vi "changeFWposAcq.vi"(0 "FW pos":u8, 1 "FWhandle":u32) -> ()   [LabVIEW 2015]
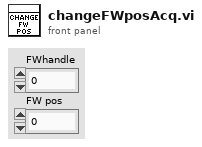
[diagram p1: front panel]
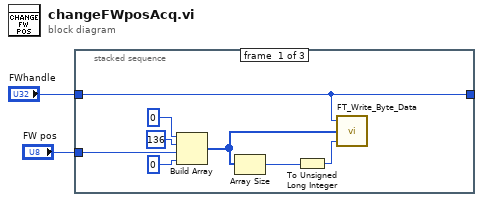
[diagram p0: block diagram]
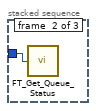
[diagram p2: hidden frame]
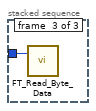
[diagram p3: hidden frame]
diagram:
  n1 = stacked-sequence {
    tunnel: "FWhandle" -> [w4 w11 w12]
    tunnel: [w4 _ _] -> _
    tunnel: "FW pos" -> [w3 _ _]
    frame #0 {
      n2 = Build Array(u8 0 ("element"), u8 136 ("element"), w3, u8 0 ("element")) -> (w10:u8[])
      n3 = Array Size(array=w10) -> (size(s)=w8:i32)
      n4 = To Unsigned Long Integer(number=w8) -> (unsigned 32bit integer=w9:u32)
      n5 = call "FT_Write_Byte_Data.vi"("Bytes To Write"=w9, "Buffer"=w10, "Handle"=w4) -> ()  [unwired: 2 out]
    }
    frame #1 {
      n6 = call "FT_Get_Queue_Status.vi"("Handle"=w11) -> ()  [unwired: 2 out]
    }
    frame #2 {
      n7 = call "FT_Read_Byte_Data.vi"("Handle"=w12) -> ()  [unwired: 1 in, 3 out]
    }
  }
